vi "Inspect Setup-Cleanup.vi"(8 "error in (no error)":errorcluster, 11 "Function":T1) -> (0 "error out":errorcluster)   [LabVIEW 2019]
uses:
  Common.llb/IVB Execution Function Code.ctl
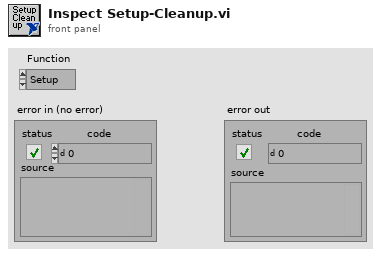
[diagram p1: front panel]
types:
  T1 = typedef "IVB Execution Function Code.ctl" = enum16{"Setup", "Exec", "Cleanup"}
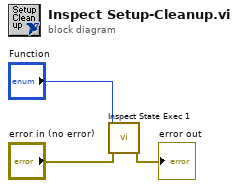
[diagram p0: block diagram]
diagram:
  n1 = call "Inspect State Exec 1.vi"("error in (no error)"="error in (no error)", "Function"="Function") -> ("error out"=→"error out":errorcluster)  [unwired: 8 in, 1 out]
